vi "参考-数组至表格字符串转换.vi"() -> ()   [LabVIEW 2018]
doc: "演示“数组至电子表格字符串转换”函数。"
panel:
  out "输出结果－电子表格字符串（'\\'代码显示）":string
  out "输出结果－电子表格字符串（正常显示）":string
  in  "格式字符串":string="%f"
  in  "分隔符（'\\'代码显示）":string="\t"
  in  "原有的二维数组":dbl[][](array[numeric])=[[0.0, 1.0, 2.0, 3.0], [4.0, 5.0, 6.0, 7.0], [8.0, 9.0, 10.0, 11.0], [12.0, 13.0, 14.0, 15.0]] format="%#.6g"
  # "概述：演示数组至电子表格字符串转换函数。\n操作步骤：\n1.运行VI。\n2.更改分隔符或格式字符串，再次运行VI后查看结果。"
  # "可对各种格式说明符进行试验，或参考帮助文档中的格式说明语法：\n%f - 带小数格式的浮点数\n%3d - 最小域宽为3个字符的带符号十进制整数\n%8.4f - 最小域宽为8个字符的浮点数。4个字符用于控制值的精度。"
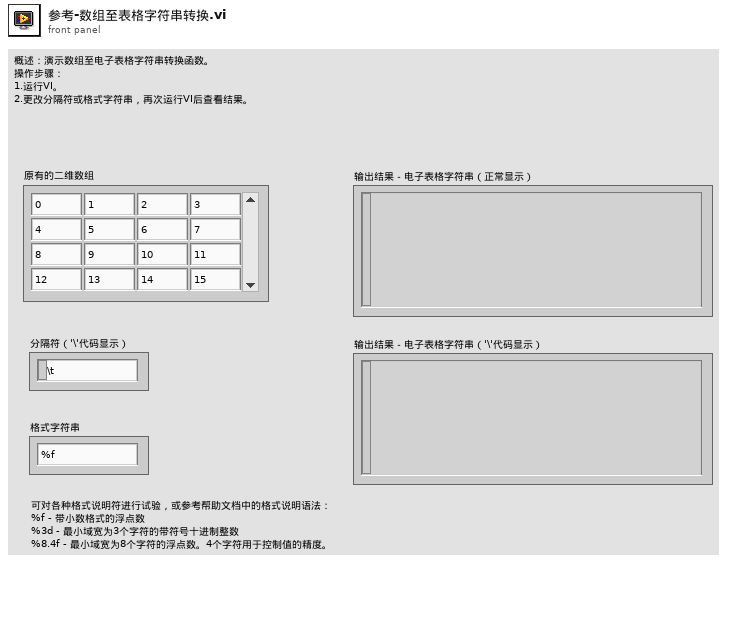
[diagram p1: front panel]
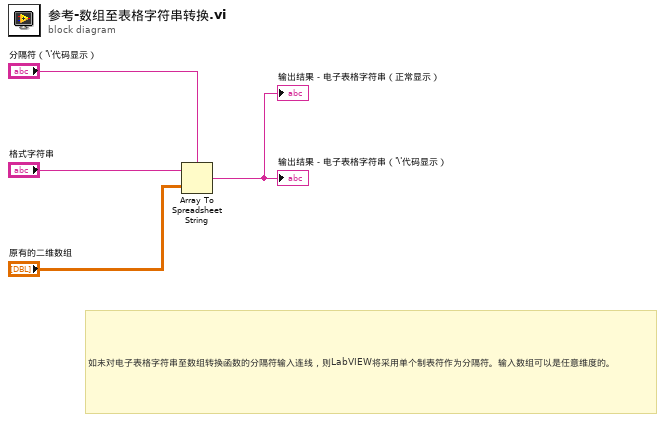
[diagram p0: block diagram]
diagram:
  # "如未对电子表格字符串至数组转换函数的分隔符输入连线，则LabVIEW将采用单个制表符作为分隔符。输入数组可以是任意维度的。"
  n1 = Array To Spreadsheet String(delimiter (Tab)="分隔符（'\\'代码显示）", array="原有的二维数组", 3:"格式字符串") -> (spreadsheet string=→"输出结果－电子表格字符串（正常显示）" →"输出结果－电子表格字符串（'\\'代码显示）":string)
